vi "Readexcel.vi"(10 "start (0, 0)":cluster{"start row":i32, "start column":i32}={"start row"=2, "start column"=1}) -> (3 "Excel设置码":string)   [LabVIEW 2020]
uses:
  <vilib>/Utility/NIReport.llb/Report Type.ctl
  <vilib>/Utility/sysdir.llb/System Directory Type.ctl
  <vilib>/addons/_office/excel.llb/Excel Get Data (str).vi
  <vilib>/Utility/NIReport.llb/NI_report.lvclass
  <vilib>/addons/_office/NI_ReportGenerationToolkit.lvlib
  <vilib>/Utility/NIReport.llb/NI_ReportGenerationCore.lvlib
  <vilib>/Utility/NIReport.llb/Excel/NI_Excel.lvclass
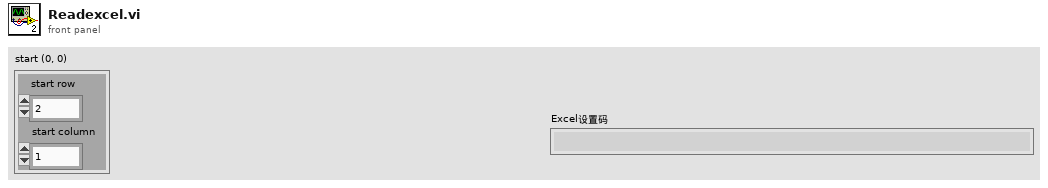
[diagram p1: front panel]
types:
  T1 = typedef "NI_ReportGenerationCore.lvlib/Report Type.ctl" = enum16{"HTML", "Word", "Excel"}
  T2 = enum16{"maximized", "minimized", "normal", "no change"}
  T3 = typedef "System Directory Type.ctl" = i32
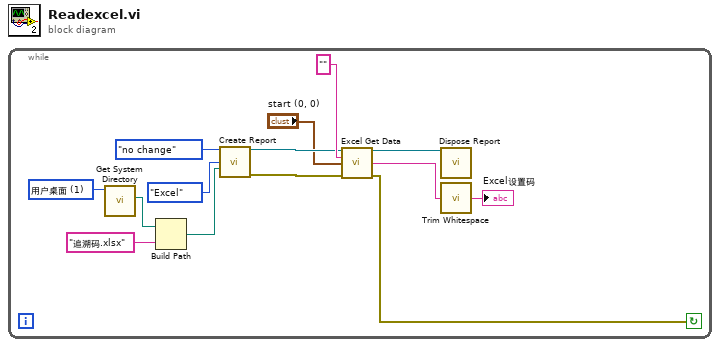
[diagram p0: block diagram]
diagram:
  n1 = while {
    stop <- w1 continue-if-true
    w8 = T3 1 items=["用户目录"=0, "用户桌面"=1, "用户文档"=2, "用户应用程序数据"=3, "用户设置"=4, "用户临时目录"=5, "公共文档"=6, "公共应用程序数据"=7, "公共设置"=8, "公共缓存"=13, "系统核心库"=9, "系统安装库"=10, "应用程序文件"=11, "启动盘根目录"=12] ("system directory type")
    n2 = call <vilib>:"Get System Directory.vi"("system directory type"=w8) -> ("system directory"=w7:path)  [unwired: 10 in]
    n3 = Build Path(base path=w7, name or relative path="追溯码.xlsx" ("名称或相对路径")) -> (appended path=w5:path)
    n4 = call <vilib>:"Create Report.vi"("window state (normal)"=T2."no change", "report type"=Report_Type."Excel", "template (empty)"=w5) -> ("report out"=w13:refnum<class "NI_report.lvclass">, "error out"=w9:errorcluster)  [unwired: 11 in]
    n5 = call-poly <vilib>:"Excel Get Data.vi"("report in"=w13, "data type"="", "start (0, 0)"="start (0, 0)", "error in (no error)"=w9) -> ("report out"=w3:refnum<class "NI_report.lvclass">, "data"=w10:string, "error out"=w1:errorcluster)  [unwired: 9 in]
    n6 = call-dynamic "Dispose Report.vi"("report in"=w3) -> ()  [unwired: 14 in, 1 out]
    n7 = call <vilib>:"Trim Whitespace.vi"("string"=w10) -> ("trimmed string"=→"Excel设置码":string)  [unwired: 1 in]
  }
